vi "Execute.vi"(8 "error in (no error)":errorcluster, 10 "System In":refnum<class "bt_System.lvclass">, 11 "Node in":refnum<class "bt_Repeat Until Timeout.lvclass">) -> (0 "error out":errorcluster, 1 "Status":T1, 2 "System Out":refnum<class "bt_System.lvclass">, 3 "Node out":refnum<class "bt_Repeat Until Timeout.lvclass">)   [LabVIEW 2021, in "BT.lvlib" / "bt_Repeat Until Timeout.lvclass"]
uses:
  bt_Repeat Until Timeout.lvclass
  abs_Node/Status.ctl
  abs_System/bt_System.lvclass
  bt_Repeat Until Timeout.lvclass/bt_Repeat Until Timeout.ctl
  Repeater/bt_Repeater.lvclass
  abs_Node/bt_Node.lvclass
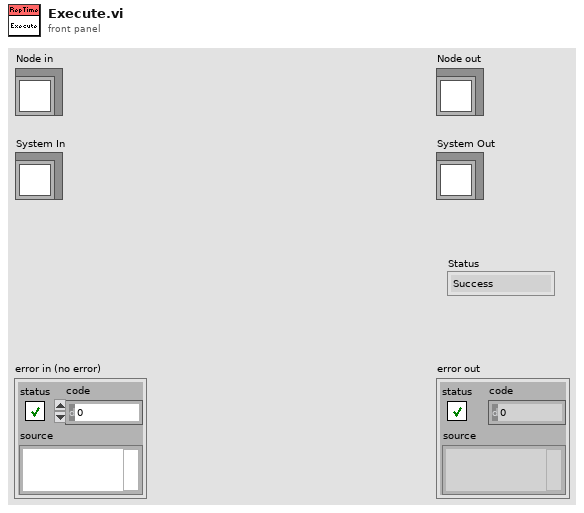
[diagram p1: front panel]
types:
  T1 = typedef "BT.lvlib/bt_Node.lvclass/Status.ctl" = enum16{"Success", "Failure", "Running"}
  T2 = typedef "BT.lvlib/bt_Repeat Until Timeout.lvclass/On Timeout Status - Type.ctl" = enum16{"Success", "Failure"}
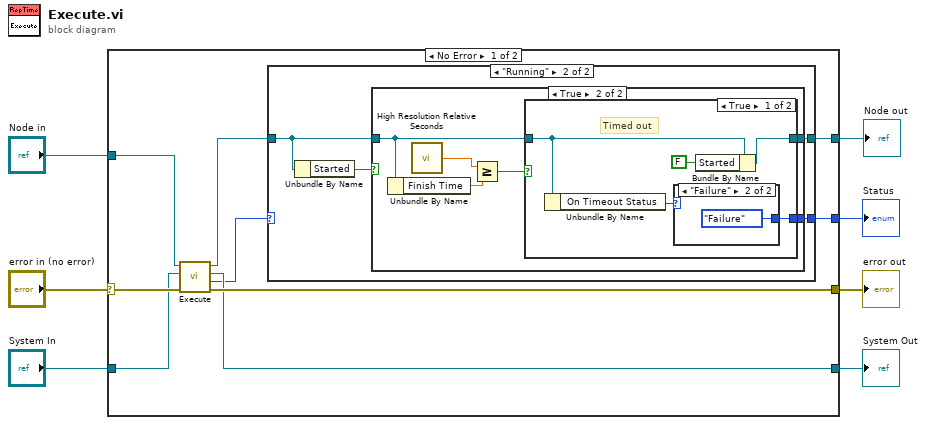
[diagram p0: block diagram]
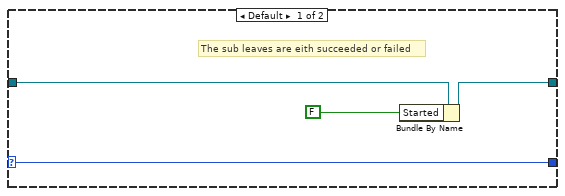
[diagram p2: hidden frame]
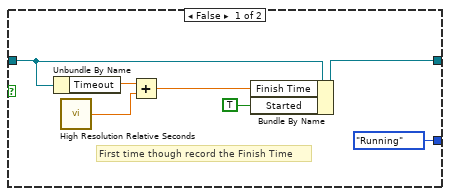
[diagram p3: hidden frame]
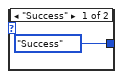
[diagram p4: hidden frame]
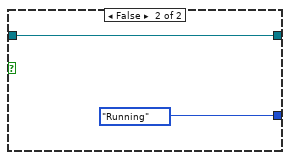
[diagram p5: hidden frame]
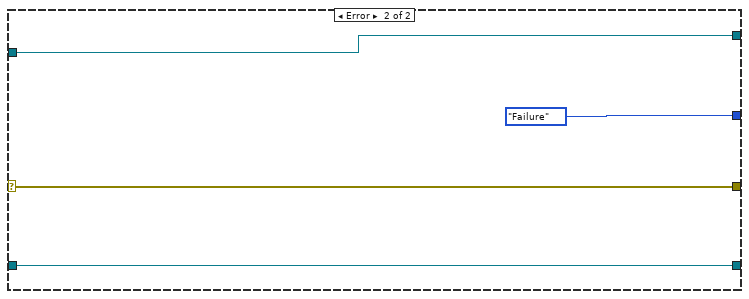
[diagram p6: hidden frame]
diagram:
  n1 = case shown="No Error" "error in (no error)" {
    selector: "error in (no error)" -> [w14 w48]
    tunnel: [w16 w48] -> w7
    tunnel: [w15 w47] -> w6
    tunnel: "System In" -> [w13 w47]
    tunnel: "Node in" -> [w12 w50]
    tunnel: [w9 Status."Failure" ("Status")] -> w2
    tunnel: [w8 w50] -> w1
    frame No Error {
      n2 = call-parent "Execute.vi"("error in (no error)"=w14, "System In"=w13, "Node in"=w12) -> ("error out"=w16:errorcluster, "Status"=w10:T1, "System Out"=w15:refnum<class "bt_System.lvclass">, "Node out"=w11:refnum<class "bt_Repeat Until Timeout.lvclass">)  [unwired: 5 in]
      n3 = case shown="\"Running\"" w10 {
        selector: w10 -> [w20 _]
        tunnel: w11 -> [w19 w22]
        tunnel: [w20 w23] -> w9
        tunnel: [w18 w24] -> w8
        frame Default {
          # "The sub leaves are eith succeeded or failed"
          n4 = Bundle By Name(cluster=w19, "Started"=FALSE) -> (w18:refnum<class "bt_Repeat Until Timeout.lvclass">)
        }
        frame "Running" {
          n5 = Unbundle By Name(w22) -> ("Started"=w21:bool)
          n6 = case shown="True" w21 {
            tunnel: w22 -> [w29 w37]
            tunnel: [w30 w36] -> w24
            tunnel: [Status."Running" ("Status") w35] -> w23
            frame False {
              # "First time though record the Finish Time"
              n7 = Unbundle By Name(w29) -> ("Timeout"=w28:dbl)
              n8 = call <vilib>:"High Resolution Relative Seconds.vi"() -> ("relative seconds"=w25:dbl)
              n9 = Add(x=w28, y=w25) -> (x+y=w27:dbl)
              n10 = Bundle By Name(cluster=w29, "Finish Time"=w27, "Started"=TRUE) -> (w30:refnum<class "bt_Repeat Until Timeout.lvclass">)
            }
            frame True {
              n11 = Unbundle By Name(w37) -> ("Finish Time"=w34:dbl)
              n12 = call <vilib>:"High Resolution Relative Seconds.vi"() -> ("relative seconds"=w33:dbl)
              n13 = Greater Or Equal?(x=w33, y=w34) -> (x >= y?=w32:bool)
              n14 = case shown="True" w32 {
                tunnel: w37 -> [w40 w46]
                tunnel: [w39 w46] -> w36
                tunnel: [w42 Status."Running" ("Status")] -> w35
                frame True {
                  # "Timed out"
                  n15 = Unbundle By Name(w40) -> ("On Timeout Status"=w41:T2)
                  n16 = case shown="\"Failure\"" w41 {
                    tunnel: [Status."Success" ("Status") Status."Failure" ("Status")] -> w42
                    frame "Success" {
                    }
                    frame "Failure" {
                    }
                  }
                  n17 = Bundle By Name(cluster=w40, "Started"=FALSE) -> (w39:refnum<class "bt_Repeat Until Timeout.lvclass">)
                }
                frame False {
                }
              }
            }
          }
        }
      }
    }
    frame Error {
    }
  }
  "error out" <- w7
  "Node out" <- w1
  "Status" <- w2
  "System Out" <- w6
